vi "Example Variant Info.vi"() -> ()   [LabVIEW 2014]
panel:
  out "variant 2":variant
  out "variant":variant
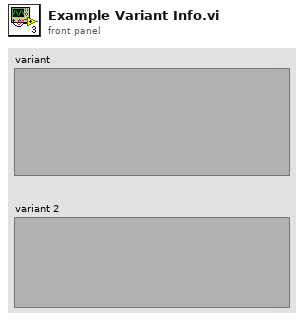
[diagram p1: front panel]
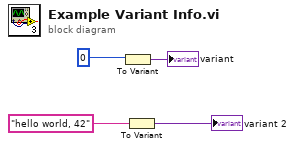
[diagram p0: block diagram]
diagram:
  n1 = To Variant(anything=0) -> (Variant=→"variant":variant)
  n2 = To Variant(anything="hello world, 42") -> (Variant=→"variant 2":variant)
